vi "test_5782_stage2.vi"() -> ()   [LabVIEW 2013]
uses:
  <vilib>/measure/maspectr.llb/Power Spectrum and PSD Export Mode.ctl
  <vilib>/measure/maspectr.llb/FFT Power Spectrum and PSD for 1 Chan (CDB).vi
  <vilib>/measure/NI_MAPro.lvlib
  <vilib>/rvi/FXPMathLib/FxpInterpret/XNode/nifxpmath_Interpret.xnode
panel:
  out "IQ data":fxp<+/-,16,14>[][](array[numeric])
  out "data out 2":dbl[][](graph)
  out "size before":i32
  out "data in":dbl[](graph)
  out "size after":i32
  out "power spectrum after":cluster{"f0":dbl, "df":dbl, "magnitude":dbl[]}(graph)
  out "power spectrum bef":cluster{"f0":dbl, "df":dbl, "magnitude":dbl[]}(graph)
  out "data out":i16[](graph)
  out "Iteration":i32
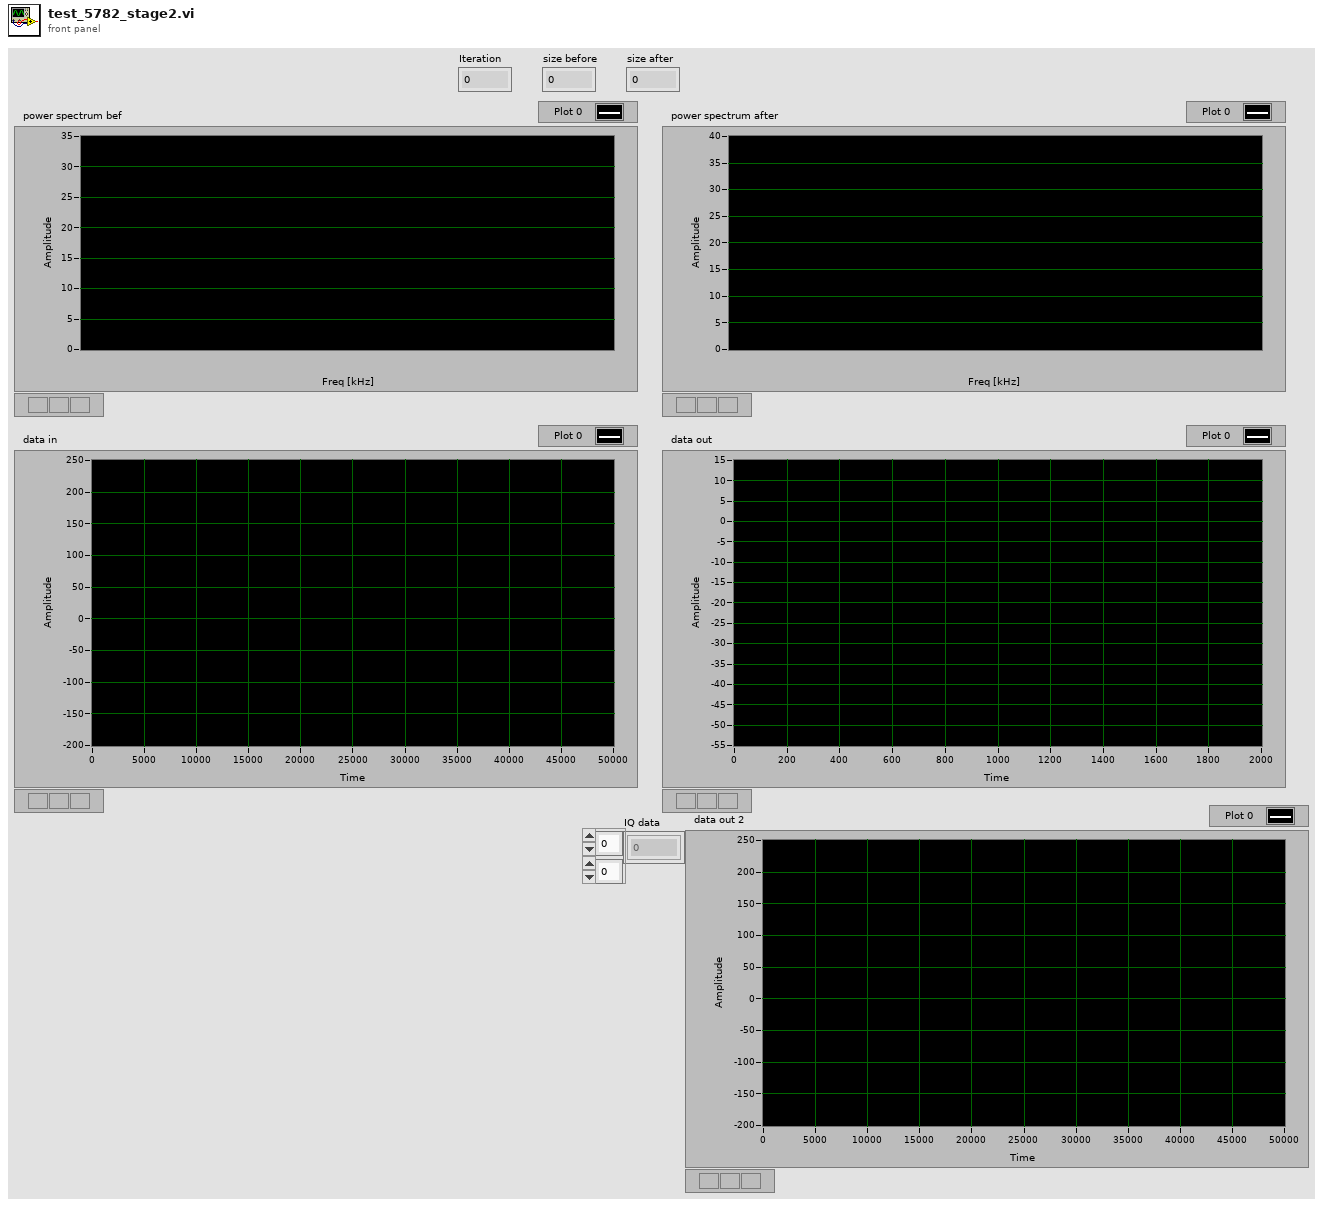
[diagram p1: front panel]
types:
  T1 = typedef "NI_MAPro.lvlib/Power Spectrum and PSD Export Mode.ctl" = u16
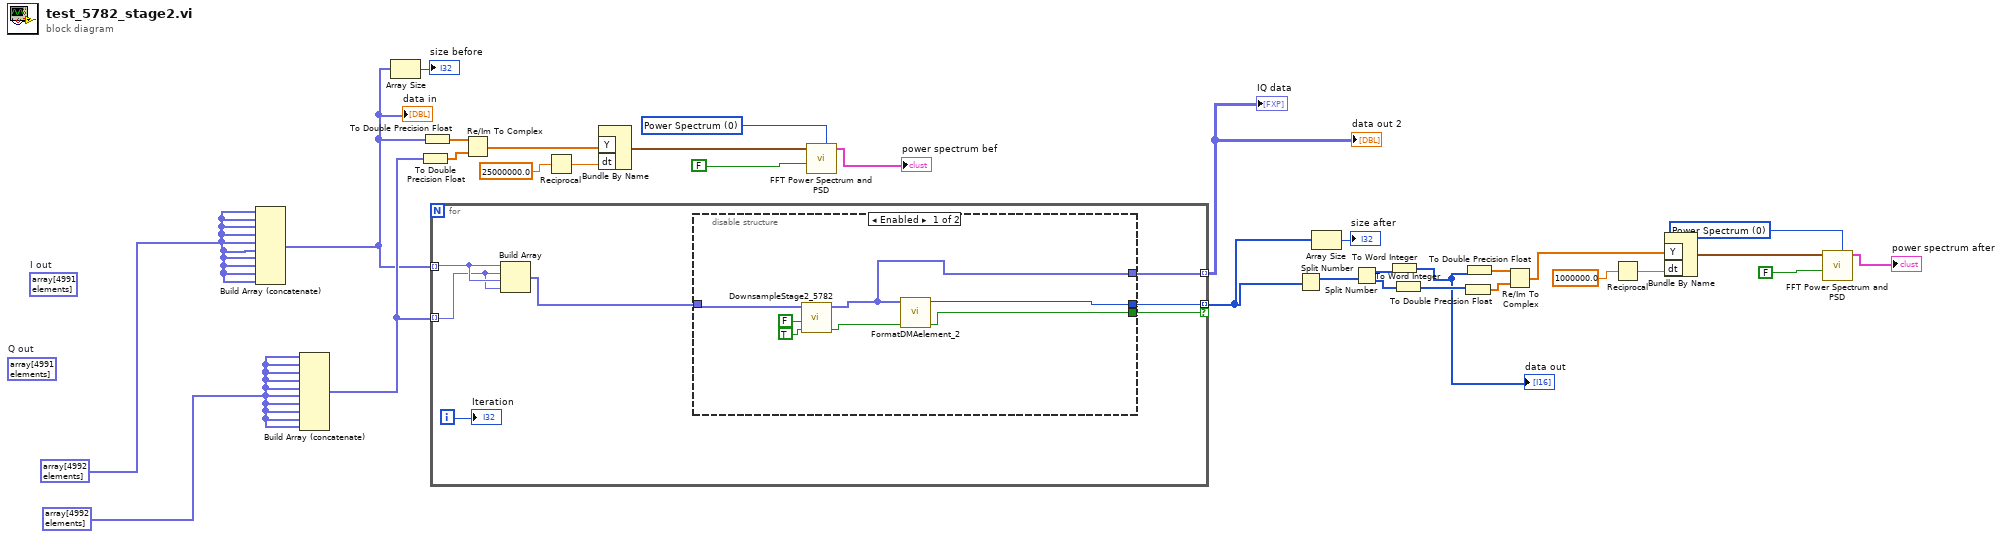
[diagram p0: block diagram]
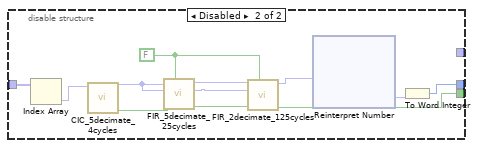
[diagram p2: hidden frame]
diagram:
  w1 = fxp<+/-,16,14>[] array[4992 elements] ("Q out")
  w2 = fxp<+/-,16,14>[] array[4992 elements] ("I out")
  (unwired) fxp<+/-,16,14>[] array[4991 elements]  # Q out
  (unwired) fxp<+/-,16,14>[] array[4991 elements]  # I out
  w17 = T1 0 items=["Power Spectrum", "Power Spectral Density"] ("export mode")
  w31 = T1 0 items=["Power Spectrum", "Power Spectral Density"] ("export mode")
  n1 = Build Array (concatenate)(w2, w2, w2, w2, w2, w2, w2, w2, w2, w2) -> (w4:fxp<+/-,16,14>[])
  "data in" <- w4
  n2 = Build Array (concatenate)(w1, w1, w1, w1, w1, w1, w1, w1, w1, w1) -> (w7:fxp<+/-,16,14>[])
  n3 = Array Size(array=w4) -> (size(s)=→"size before":i32)
  n4 = To Double Precision Float(number=w7) -> (double precision float=w24:dbl[])
  n5 = To Double Precision Float(number=w4) -> (double precision float=w25:dbl[])
  n6 = for {
    tunnel: w4 -> [w38] mode=indexing
    tunnel: w7 -> [w37] mode=indexing
    tunnel: [w34] -> w6 mode=indexing if=w32
    tunnel: [w33] -> w3 mode=indexing
    i -> [w36]
    n7 = Build Array(w38, w37, w38, w37) -> (w35:fxp<+/-,16,14>[])
    n8 = disable-structure shown="Enabled" {
      disable-tunnel: w35 -> [w44 w52]
      disable-tunnel: [w40 w50] -> w32
      disable-tunnel: [w42 w47] -> w34
      disable-tunnel: [w39 _] -> w33
      frame Enabled {
        n9 = call "DownsampleStage2_5782.vi"("valid in"=TRUE, "reset"=FALSE, "Data in"=w44) -> ("valid out"=w41:bool, "data out"=w39:fxp<+/-,16,14>[])  [unwired: 7 in]
        n10 = call "FormatDMAelement_2.vi"("valid in"=w41, "Data in"=w39) -> ("valid out"=w40:bool, "Element1"=w42:u64)  [unwired: 8 in]
      }
      frame Disabled {
        w54 = FALSE ("reset")
        n11 = Index Array(array=w52) -> (element=w51:fxp<+/-,16,14>)  [unwired: 1 in]
        n12 = call "CIC_5decimate_4cycles.vi"("Data in"=w51) -> ("valid out"=w57:bool, "Data out"=w58:fxp<+/-,16,14>, "valid in"=w46:bool)  [unwired: 7 in, 1 out]
        n13 = call "FIR_5decimate_25cycles.vi"("reset"=w54, "valid in"=w57, "Q in"=w58, "I in"=w58) -> ("valid out"=w53:bool, "Q out"=w55:fxp<+/-,16,14>, "I out"=w56:fxp<+/-,16,14>)  [unwired: 4 in, 1 out]
        n14 = call "FIR_2decimate_125cycles.vi"("reset"=w54, "valid in"=w53, "Q in"=w55, "I in"=w56) -> ("valid out"=w50:bool, "I out"=w48:fxp<+/-,16,14>)  [unwired: 4 in, 2 out]
        n15 = xnode "Reinterpret Number"("x"=w48) -> ("y"=w49:fxp<+/-,16,16>)
        n16 = To Word Integer(number=w49) -> (16bit integer=w47:i16)
      }
    }
    "Iteration" <- w36
  }
  "data out 2" <- w3
  "IQ data" <- w3
  n17 = Re/Im To Complex(1:w24, 2:w25) -> (0:w23:cdb[])
  n18 = Reciprocal(x=25000000.0 ("dt")) -> (1/x=w27:dbl)
  n19 = Bundle By Name("Y"=w23, "dt"=w27) -> (w30:waveform(cdb))  [unwired: 1 in]
  n20 = call-poly <vilib>:"FFT Power Spectrum and PSD.vi"("export mode"=w31, "dB On (F)"=FALSE, "time signal"=w30) -> ("Power Spectrum / PSD"=→"power spectrum bef":cluster{"f0":dbl, "df":dbl, "magnitude":dbl[]})  [unwired: 5 in, 3 out]
  n21 = Split Number(x=w6) -> (hi(x)=w13:u32[])  [unwired: 1 out]
  n22 = Array Size(array=w6) -> (size(s)=→"size after":i32)
  n23 = Split Number(x=w13) -> (hi(x)=w12:u16[], lo(x)=w11:u16[])
  n24 = To Word Integer(number=w12) -> (16bit integer=w9:i16[])
  "data out" <- w9
  n25 = To Word Integer(number=w11) -> (16bit integer=w10:i16[])
  n26 = To Double Precision Float(number=w10) -> (double precision float=w16:dbl[])
  n27 = To Double Precision Float(number=w9) -> (double precision float=w15:dbl[])
  n28 = Re/Im To Complex(1:w16, 2:w15) -> (0:w14:cdb[])
  n29 = Reciprocal(x=1000000.0 ("dt")) -> (1/x=w21:dbl)
  n30 = Bundle By Name("Y"=w14, "dt"=w21) -> (w18:waveform(cdb))  [unwired: 1 in]
  n31 = call-poly <vilib>:"FFT Power Spectrum and PSD.vi"("export mode"=w17, "dB On (F)"=FALSE, "time signal"=w18) -> ("Power Spectrum / PSD"=→"power spectrum after":cluster{"f0":dbl, "df":dbl, "magnitude":dbl[]})  [unwired: 5 in, 3 out]
